vi "Begin.vi"() -> (0 "error out":errorcluster)   [LabVIEW 2013]
doc: "Called before other user functions, this VI is expected to open initial I/O refnums, load in file data, and do all program initialization. Notice that the <B>error out</B> terminal is simply used for data flow. Wiring it to other structures or subVIs ensures that this VI runs first."
uses:
  <vilib>/Rock Robotics/SystemInterfaces/DIO/FPGA_DIOPWMChannel.ctl
  <vilib>/Rock Robotics/WPI/SafetyOutput/WPI_SafetyOutputConfigMenu.ctl
  <vilib>/Rock Robotics/WPI/DriverStation/WPI_DriverStationRobotMode2.ctl
  <vilib>/Rock Robotics/WPI/Joystick/WPI_JoystickDeviceEnum.ctl
  <vilib>/Rock Robotics/SystemInterfaces/DIO/FPGA_DIORelayChannel.ctl
  <vilib>/Rock Robotics/SystemInterfaces/DIO/FPGA_DIOChannel.ctl
  <vilib>/Rock Robotics/SystemInterfaces/Typedef/FPGA_TypedefDigitalModule.ctl
  <vilib>/Rock Robotics/WPI/Solenoid/WPI_SolenoidChannel.ctl
  TankDriveAction.ctl
  QueueAction.ctl
  <vilib>/Rock Robotics/SystemInterfaces/Typedef/FPGA_TypedefSolenoidModule.ctl
  <vilib>/Rock Robotics/WPI/RobotDrive/WPI_RobotDriveOpen2MotorWithTalon.vi
  Robot Global Data.vi
  OutputError.vi
  OutputErrors.vi
  <vilib>/Rock Robotics/WPI/Solenoid/WPI_SolenoidOpenSingle.vi
  <vilib>/Rock Robotics/WPI/Compressor/WPI_CompressorGetSetRefNum.vi
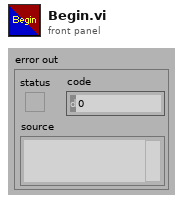
[diagram p1: front panel]
types:
  T1 = typedef "WPI_SolenoidChannel.ctl" = enum8{"Solenoid 1", "Solenoid 2", "Solenoid 3", "Solenoid 4", "Solenoid 5", "Solenoid 6", "Solenoid 7", "Solenoid 8", "Invalid"}
  T2 = typedef "FPGA_TypedefSolenoidModule.ctl" = enum16{"Solenoid Module 1", "Solenoid Module 2"}
  T3 = typedef "QueueAction.ctl" = enum16{"Init", "SetValue", "Disable"}
  T4 = typedef "TankDriveAction.ctl" = enum16{"Init", "LinearDrive", "SetValue", "Disable"}
  T5 = typedef "WPI_JoystickDeviceEnum.ctl" = enum16{"USB 1", "USB 2", "USB 3", "USB 4", "Kinect 1", "Kinect 2"}
  T6 = typedef "FPGA_TypedefDigitalModule.ctl" = enum16{"Digital Module 1", "Digital Module 2"}
  T7 = typedef "FPGA_DIOChannel.ctl" = enum8{"DIO 1", "DIO 2", "DIO 3", "DIO 4", "DIO 5", "DIO 6", "DIO 7", "DIO 8", "DIO 9", "DIO 10", "DIO 11", "DIO 12", "DIO 13", "DIO 14", "Invalid"}
  T8 = typedef "FPGA_DIORelayChannel.ctl" = enum8{"Relay 1", "Relay 2", "Relay 3", "Relay 4", "Relay 5", "Relay 6", "Relay 7", "Relay 8", "Invalid"}
  T9 = typedef "WPI_DriverStationRobotMode2.ctl" = enum16{"Autonomous Disabled", "Autonomous Enabled", "Teleop Disabled", "Teleop Enabled", "Timeout", "Finish", "Test Disabled", "Test Enabled"}
  T10 = typedef "WPI_SafetyOutputConfigMenu.ctl" = enum16{"Enable", "Disable"}
  T11 = typedef "FPGA_DIOPWMChannel.ctl" = enum8{"PWM 1", "PWM 2", "PWM 3", "PWM 4", "PWM 5", "PWM 6", "PWM 7", "PWM 8", "PWM 9", "PWM 10", "Invalid"}
  T12 = typedef "WPI_JoystickDevRef.ctl" = cluster{"Device":T5}
  T13 = typedef "WPI_RobotDriveDevRef.ctl" = cluster{"DevStatus":errorcluster, "Motors[]":T14[], "Square Inputs":bool, "Max Output":dbl, "Isochronous":bool}
  T14 = typedef "WPI_MotorControlDeviceRef.ctl" = cluster{"DeviceStatus":errorcluster, "Type":enum16{"PWM", "CAN"}, "PWM":cluster{"Digital Module":T6, "PWM Channel":T11, "DeadBand":T15}, "CAN":cluster{"Device Number":u8, "Control Mode":T16, "Semaphore":T17, "Max Vout":dbl}, "Invert":bool, "TransformRef":T18, "InvTransformRef":T18}
  T15 = typedef "WPI_PWMDeadband.ctl" = cluster{"Name":string, "maxPositivePwm":i32, "minPositivePwm":i32, "centerPwm":i32, "maxNegativePwm":i32, "minNegativePwm":i32, "angularRange":u16}
  T16 = typedef "WPI_CANJaguar_ControlMode.ctl" = enum8{"Percent VBus", "Current", "Speed", "Position", "Voltage"}
  T17 = typedef "Semaphore RefNum" = refnum<k1>
  T18 = typedef "WPI_PWMTransform_ConPane.ctl" = refnum<vi>
  T19 = typedef "WPI_CompressorDevRef.ctl" = cluster{"DevStatus":errorcluster, "DigitalInputDevRef":T20, "RelayDevRef":T21}
  T20 = typedef "WPI_DigitalInputDevRef.ctl" = cluster{"DevStatus":errorcluster, "DIO Channel":T7, "Digital Module":T6}
  T21 = typedef "WPI_RelayDevRef.ctl" = cluster{"DevStatus":errorcluster, "Relay Channel":T8, "Digital Module":T6, "Relay Direction":T22}
  T22 = typedef "WPI_RelayDirection.ctl" = enum16{"Both directions", "Forward only", "Reverse only"}
  T23 = typedef "WPI_SolenoidDevRef.ctl" = cluster{"DevStatus":errorcluster, "Solenoid Module":T2, "Forward Solenoid Channel":T1, "Reverse Solenoid Channel":T1}
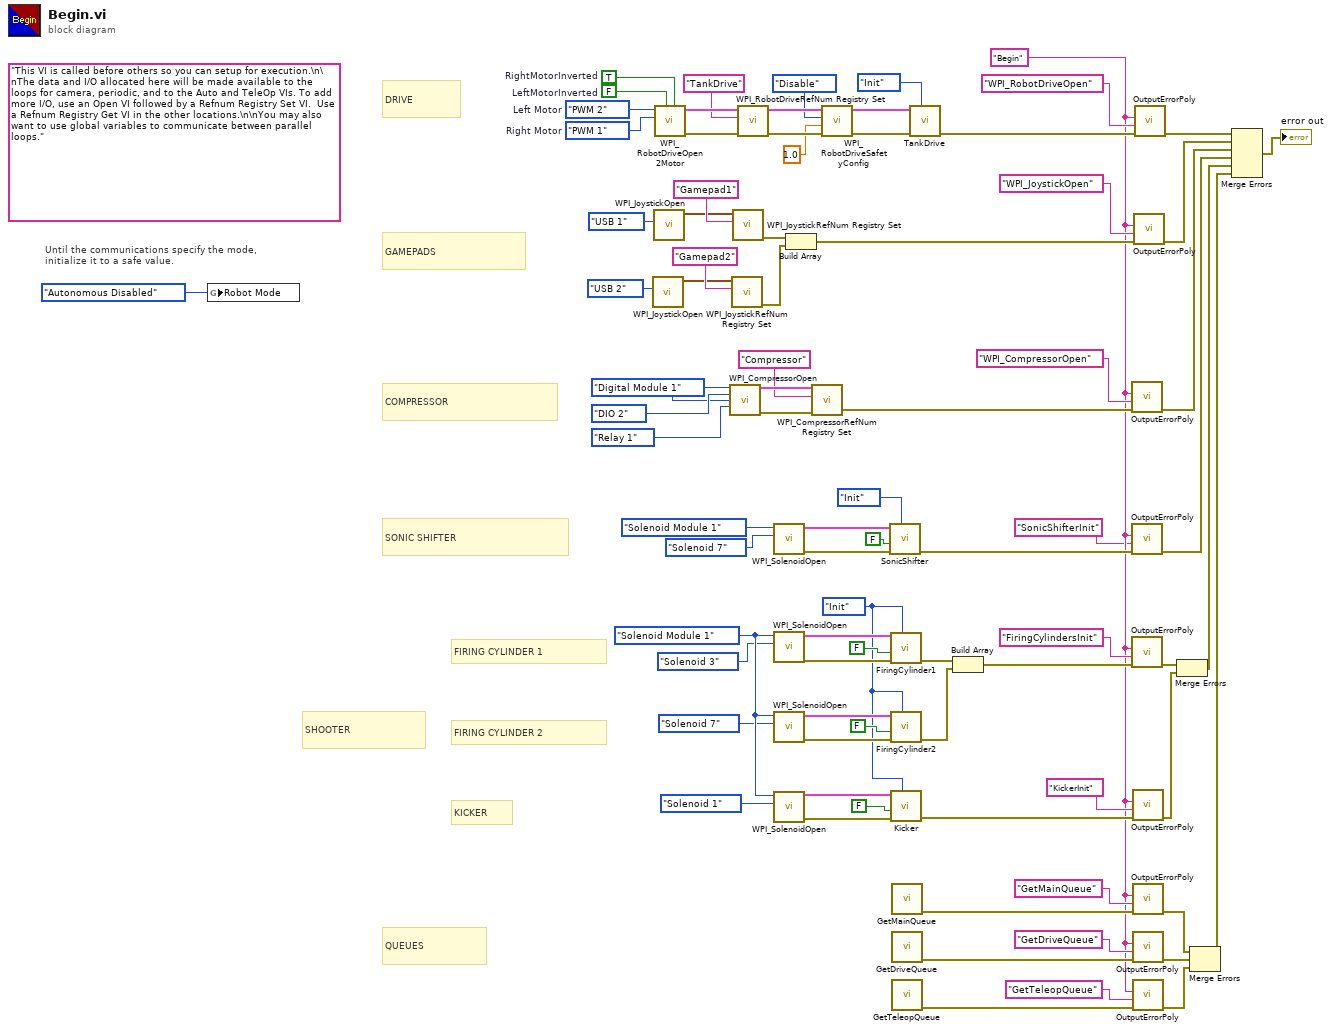
[diagram p0: block diagram]
diagram:
  w37 = FPGA_TypedefSolenoidModule."Solenoid Module 1" ("Solenoid Module (Module 1)")
  w11 = QueueAction."Init" ("Action")
  w59 = FPGA_TypedefDigitalModule."Digital Module 1" ("Pressure Switch\nand Relay Module")
  w3 = "Begin"
  (unwired) "This VI is called before others so you can setup for execution.\n\nThe data and I/O allocated here will be made available to the loops for camera, periodic, and to the Auto and TeleOp VIs. To add more I/O, use an Open VI followed by a Refnum Registry Set VI.  Use a Refnum Registry Get VI in the other locations.\n\nYou may also want to use global variables to communicate between parallel loops."
  w76 = FPGA_DIOPWMChannel."PWM 1"  # Right Motor
  w77 = FPGA_DIOPWMChannel."PWM 2"  # Left Motor
  w81 = FALSE  # LeftMotorInverted
  w82 = TRUE  # RightMotorInverted
  # "SONIC SHIFTER"
  # "QUEUES"
  # "KICKER"
  # "FIRING CYLINDER 2"
  # "FIRING CYLINDER 1"
  # "SHOOTER"
  # "COMPRESSOR"
  # "GAMEPADS"
  # "DRIVE"
  # "Until the communications specify the mode,\ninitialize it to a safe value."
  n1 = global write "Robot Global Data.vi" "Robot Mode"(WPI_DriverStationRobotMode2."Autonomous Disabled" ("Robot Mode")) -> ()
  n2 = call <vilib>:"WPI_JoystickOpen.vi"("JoystickDevice"=WPI_JoystickDeviceEnum."USB 2") -> ("JoystickDevRef"=w55:T12)  [unwired: 10 in]
  n3 = call <vilib>:"WPI_JoystickOpen.vi"("JoystickDevice"=WPI_JoystickDeviceEnum."USB 1") -> ("JoystickDevRef"=w71:T12)  [unwired: 10 in]
  n4 = call-poly <vilib>:"WPI_RobotDriveOpen2Motor.vi"("Right Motor Inverted"=w82, "Left Motor Inverted"=w81, "Right Motor"=w76, "Left Motor"=w77) -> ("error out"=w78:errorcluster, "RobotDriveDevRef"=w80:T13)  [unwired: 1 in, 5 out]
  n5 = call <vilib>:"WPI_CompressorOpen.vi"("Pressure Switch Digital Module (Module 1)"=w59, "Pressure Switch DIO Channel"=FPGA_DIOChannel."DIO 2" ("Pressure Switch Channel"), "Relay Digital Module (Module 1)"=w59, "Relay Channel"=FPGA_DIORelayChannel."Relay 1") -> ("CompressorDevRef"=w63:T19, "error out"=w61:errorcluster)  [unwired: 1 in, 9 out]
  n6 = call <vilib>:"WPI_JoystickRefNum Registry Set.vi"("refnum name"="Gamepad2", "JoystickDevRef"=w55) -> ("error out"=w52:errorcluster)  [unwired: 8 in, 1 out]
  n7 = call <vilib>:"WPI_JoystickRefNum Registry Set.vi"("refnum name"="Gamepad1", "JoystickDevRef"=w71) -> ("error out"=w53:errorcluster)  [unwired: 8 in, 1 out]
  n8 = call <vilib>:"WPI_RobotDriveRefNum Registry Set.vi"("error in (no error)"=w78, "refnum name"="TankDrive", "RobotDriveDevRef"=w80) -> ("error out"=w69:errorcluster, "RobotDriveDevRef"=w75:T13)  [unwired: 7 out]
  n9 = call-poly <vilib>:"WPI_SolenoidOpen.vi"("Solenoid Channel"=WPI_SolenoidChannel."Solenoid 7", "Solenoid Module (Module 1)"=FPGA_TypedefSolenoidModule."Solenoid Module 1") -> ("error out"=w7:errorcluster, "SolenoidDevRef"=w8:T23)  [unwired: 8 in]
  n10 = call-poly <vilib>:"WPI_SolenoidOpen.vi"("Solenoid Channel"=WPI_SolenoidChannel."Solenoid 3", "Solenoid Module (Module 1)"=w37) -> ("error out"=w40:errorcluster, "SolenoidDevRef"=w43:T23)  [unwired: 8 in]
  n11 = call-poly <vilib>:"WPI_SolenoidOpen.vi"("Solenoid Channel"=WPI_SolenoidChannel."Solenoid 7", "Solenoid Module (Module 1)"=w37) -> ("error out"=w42:errorcluster, "SolenoidDevRef"=w39:T23)  [unwired: 8 in]
  n12 = call-poly <vilib>:"WPI_SolenoidOpen.vi"("Solenoid Channel"=WPI_SolenoidChannel."Solenoid 1", "Solenoid Module (Module 1)"=w37) -> ("error out"=w41:errorcluster, "SolenoidDevRef"=w38:T23)  [unwired: 8 in]
  n13 = Build Array(w53, w52) -> (w51:errorcluster[])
  n14 = call <vilib>:"WPI_CompressorRefNum Registry Set.vi"("error in (no error)"=w61, "refnum name"="Compressor", "CompressorDevRef"=w63) -> ("error out"=w58:errorcluster)  [unwired: 7 in, 1 out]
  n15 = call <vilib>:"WPI_RobotDriveSafetyConfig.vi"("error in (no error)"=w69, "timeout (s)"=1.0, "mode"=WPI_SafetyOutputConfigMenu."Disable", "RobotDriveDevRef"=w75) -> ("error out"=w23:errorcluster, "RobotDriveDevRef"=w24:T13)  [unwired: 6 in]
  n16 = call "SonicShifter.vi"("Action"=QueueAction."Init", "error in (no error)"=w7, "Default Position"=FALSE, "SolenoidDevRef"=w8) -> ("error out"=w4:errorcluster)  [unwired: 7 in]
  n17 = call "FiringCylinder1.vi"("Action"=w11, "error in (no error)"=w40, "Default Position"=FALSE, "SolenoidDevRef"=w43) -> ("error out"=w45:errorcluster)  [unwired: 7 in]
  n18 = call "FiringCylinder2.vi"("Action"=w11, "error in (no error)"=w42, "Default Position"=FALSE, "SolenoidDevRef"=w39) -> ("error out"=w46:errorcluster)  [unwired: 7 in]
  n19 = call "Kicker.vi"("Action"=w11, "error in (no error)"=w41, "Default Position"=FALSE, "SolenoidDevRef"=w38) -> ("error out"=w47:errorcluster)  [unwired: 7 in]
  n20 = call "GetMainQueue.vi"() -> ("error out"=w21:errorcluster)  [unwired: 10 in, 1 out]
  n21 = call "GetDriveQueue.vi"() -> ("error out"=w20:errorcluster)  [unwired: 10 in, 1 out]
  n22 = call "GetTeleopQueue.vi"() -> ("error out"=w19:errorcluster)  [unwired: 10 in, 1 out]
  n23 = call "TankDrive.vi"("DriveAction"=TankDriveAction."Init", "error in (no error)"=w23, "RobotDriveDevRef"=w24) -> ("error out"=w22:errorcluster)  [unwired: 8 in]
  n24 = Build Array(w45, w46) -> (w44:errorcluster[])
  n25 = call-poly "OutputErrorPoly.vi"("error in (no error)"=w58, "Causing VI"="WPI_CompressorOpen" ("Calling VI"), "Calling VI"=w3) -> ("error out"=w48:errorcluster)  [unwired: 8 in]
  n26 = call-poly "OutputErrorPoly.vi"("error in (no error)"=w4, "Causing VI"="SonicShifterInit", "Calling VI"=w3) -> ("error out"=w1:errorcluster)  [unwired: 8 in]
  n27 = call-poly "OutputErrorPoly.vi"("errors in"=w44, "Causing VI"="FiringCylindersInit", "Calling VI"=w3) -> ("error out"=w33:errorcluster)  [unwired: 8 in]
  n28 = call-poly "OutputErrorPoly.vi"("error in (no error)"=w47, "Causing VI"="KickerInit", "Calling VI"=w3) -> ("error out"=w32:errorcluster)  [unwired: 8 in]
  n29 = call-poly "OutputErrorPoly.vi"("error in (no error)"=w21, "Causing VI"="GetMainQueue", "Calling VI"=w3) -> ("error out"=w16:errorcluster)  [unwired: 8 in]
  n30 = call-poly "OutputErrorPoly.vi"("error in (no error)"=w20, "Causing VI"="GetDriveQueue", "Calling VI"=w3) -> ("error out"=w17:errorcluster)  [unwired: 8 in]
  n31 = call-poly "OutputErrorPoly.vi"("error in (no error)"=w19, "Causing VI"="GetTeleopQueue", "Calling VI"=w3) -> ("error out"=w18:errorcluster)  [unwired: 8 in]
  n32 = call-poly "OutputErrorPoly.vi"("errors in"=w51, "Causing VI"="WPI_JoystickOpen", "Calling VI"=w3) -> ("error out"=w50:errorcluster)  [unwired: 8 in]
  n33 = call-poly "OutputErrorPoly.vi"("error in (no error)"=w22, "Causing VI"="WPI_RobotDriveOpen", "Calling VI"=w3) -> ("error out"=w49:errorcluster)  [unwired: 8 in]
  n34 = Merge Errors(w33, w32) -> (w31:errorcluster)
  n35 = Merge Errors(w16, w17, w18) -> (w15:errorcluster)
  n36 = Merge Errors(w49, w50, w48, w1, w31, w15) -> (→"error out":errorcluster)
